vi "Trim Empty Value.vi"(11 "Data In":string[](array[string])) -> (3 "Data Out":string[](array[string]))   [LabVIEW 2021, in "User Interface.lvlib"]
uses:
  User Interface.lvlib
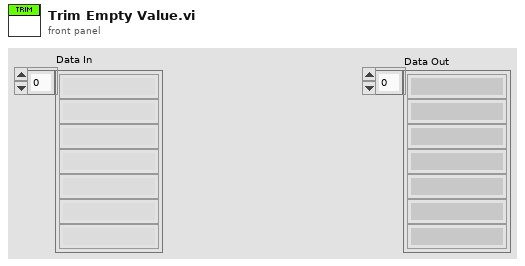
[diagram p1: front panel]
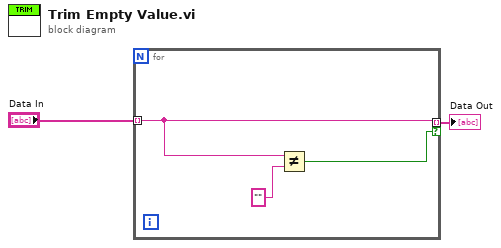
[diagram p0: block diagram]
diagram:
  n1 = for {
    tunnel: "Data In" -> [w4] mode=indexing
    tunnel: [w4] -> w1 mode=indexing if=w3
    n2 = Not Equal?(x=w4, y="") -> (x != y?=w3:bool)
  }
  "Data Out" <- w1
